vi "task_default.vi"() -> ()   [LabVIEW 2015]
uses:
  Framework/pdbm_test_route/UsrDefine/TaskFeedbackCmd.ctl
  Framework/pdbm_test_route/UsrDefine/TaskReqst.ctl
  Framework/pdbm_tasks/pdbm_tasks.lvlib
  Framework/pdbm_test_route/pdbm_task_route.lvlib
panel:
  in  "error in (no error)":errorcluster
  in  "pdbm_task_data":T1
  # "IMT APPLICATION TASK"
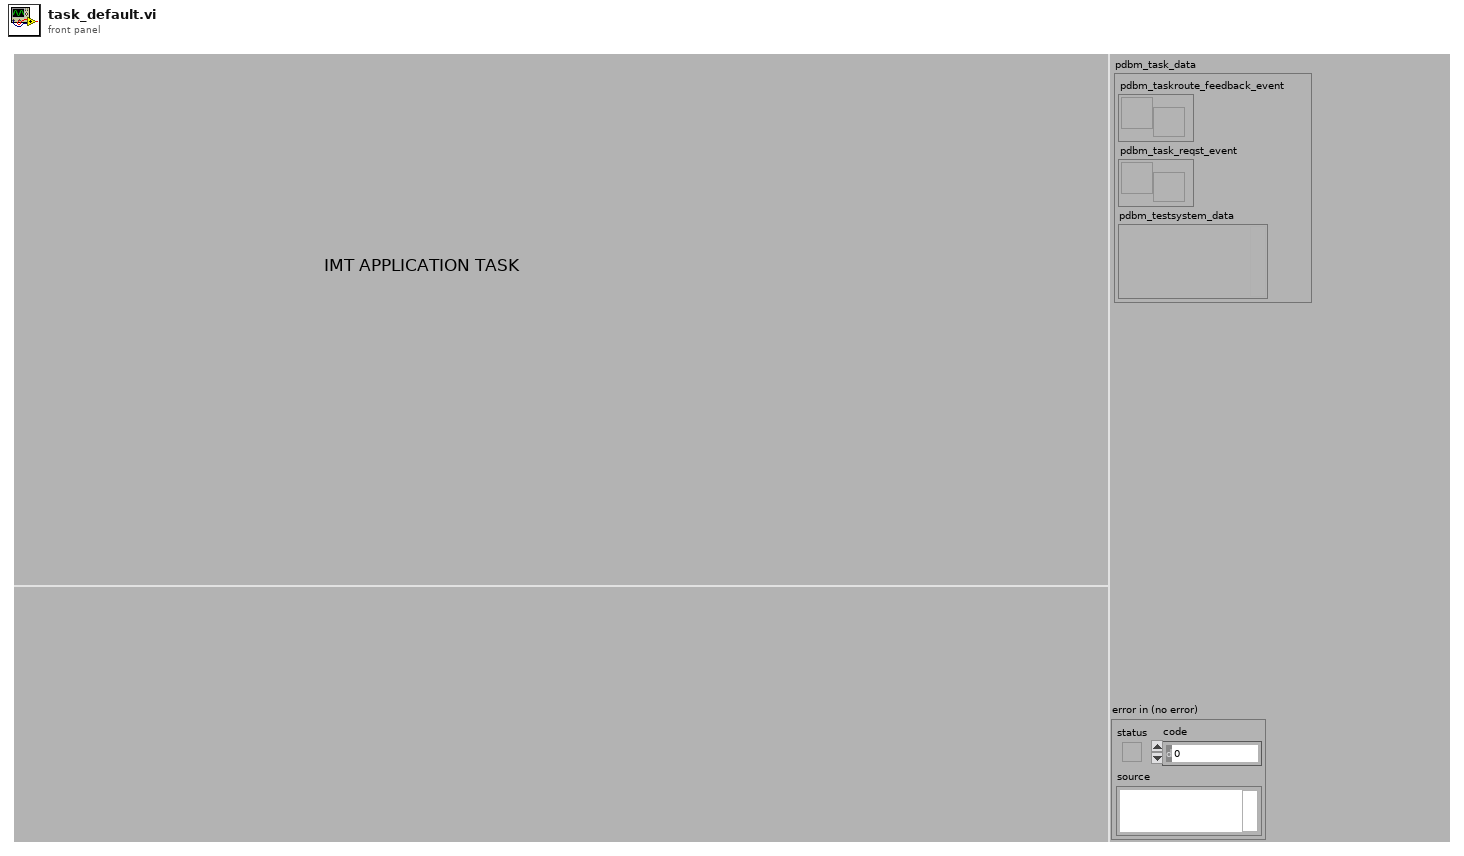
[diagram p1: front panel]
types:
  T1 = cluster{"pdbm_taskroute_feedback_event":refnum<user-event>, "pdbm_task_reqst_event":refnum<user-event>, "pdbm_testsystem_data":variant}
  T2 = typedef "pdbm_tasks.lvlib/PDBM_TestSystem_Data.ctl" = cluster{"pdbm_general_report_info":refnum<vi>, "pdbm_task_progress":refnum<vi>, "pdbm_TestButton":refnum<vi>}
  T3 = cluster{"pdbm_task_reqst_event":refnum<user-event>, "pdbm_taskroute_feedback_event":refnum<user-event>}
  T4 = typedef "pdbm_tasks.lvlib/TaskRequest.ctl" = cluster{"Command":string, "Variant":variant}
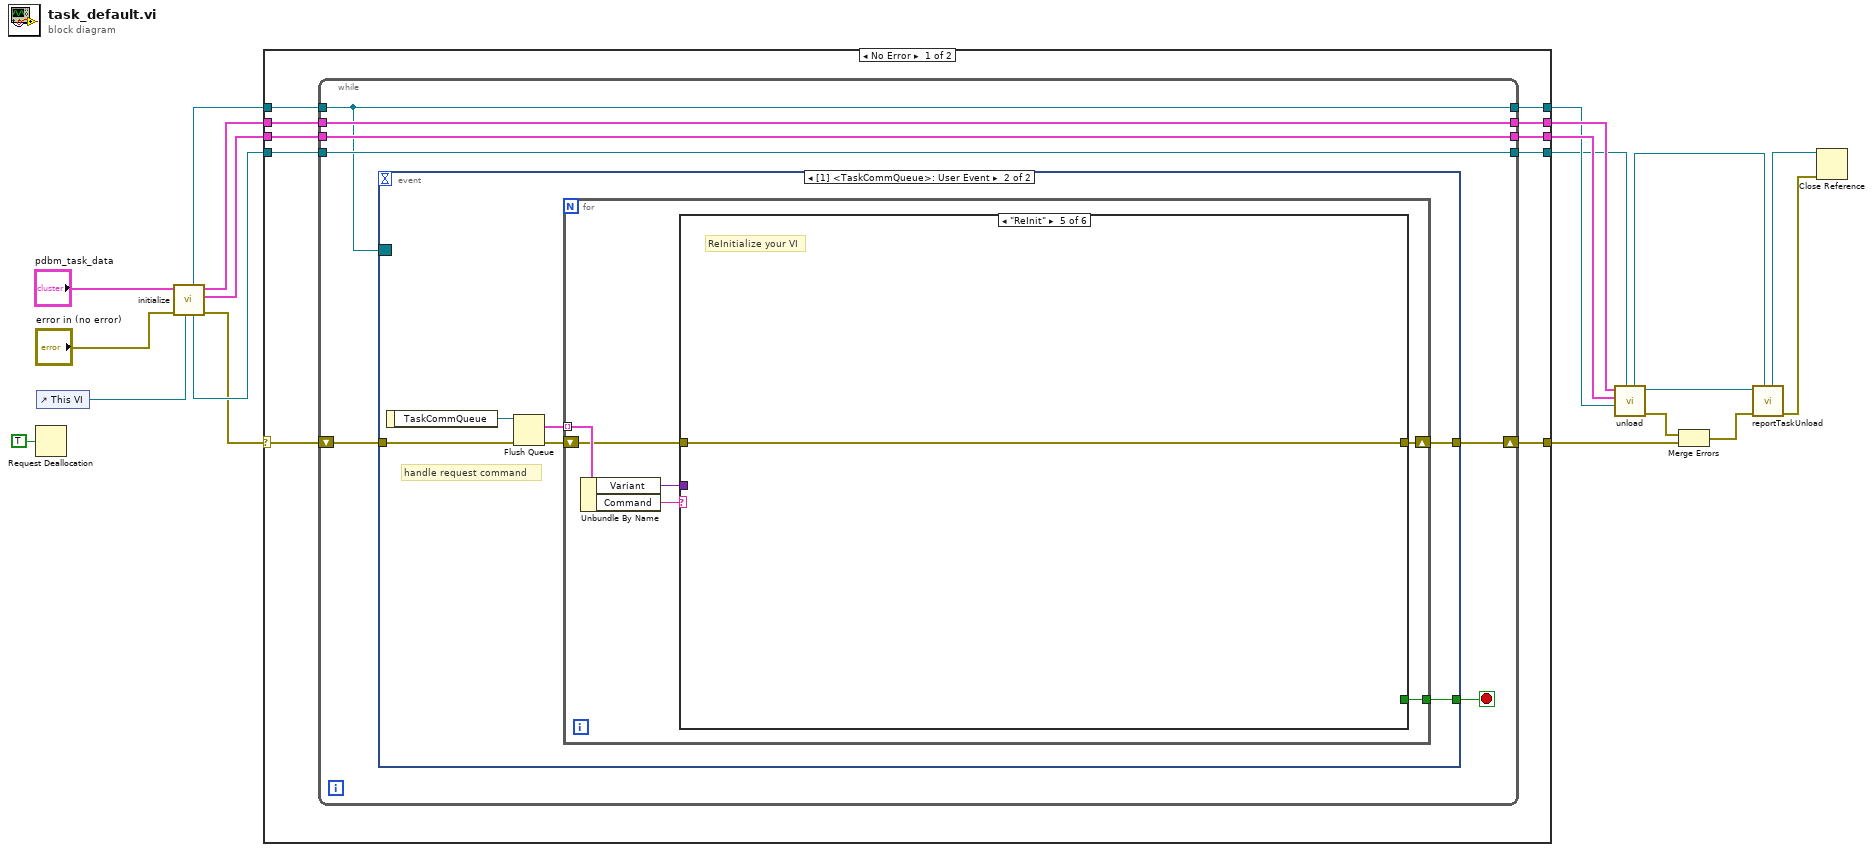
[diagram p0: block diagram]
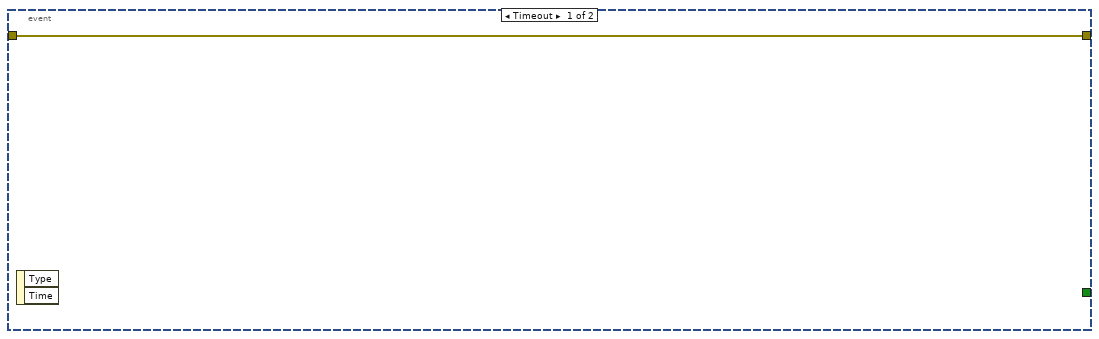
[diagram p2: hidden frame]
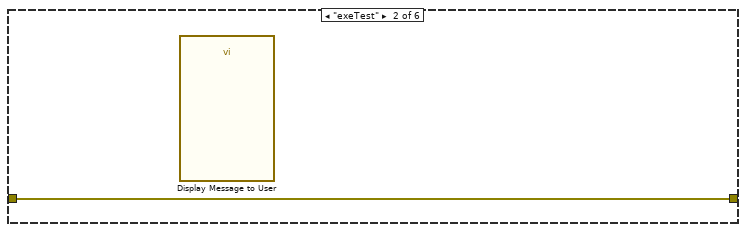
[diagram p4: hidden frame]
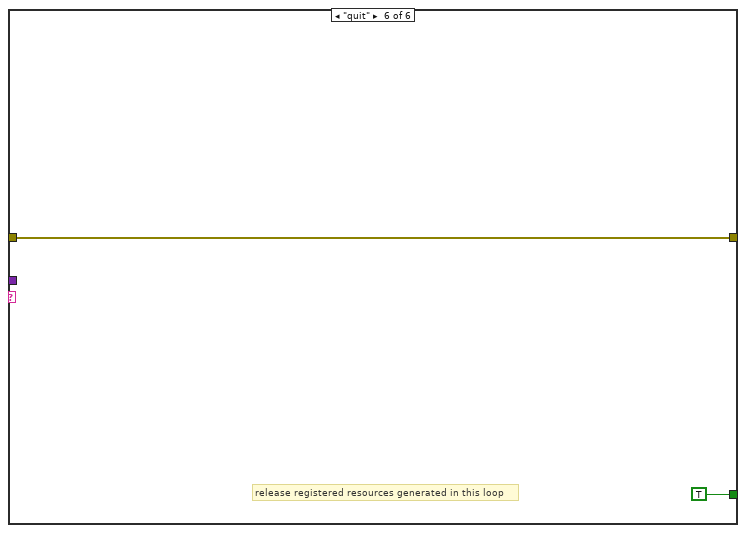
[diagram p7: hidden frame]
diagram:
  n1 = Request Deallocation(TRUE ("flag")) -> ()
  n2 = control-ref of="This VI"() -> (w19:refnum<vi>)
  n3 = call "initialize.vi"("TaskRef in"=w19, "error in"="error in (no error)", "pdbm_task_data"="pdbm_task_data") -> ("error out"=w15:errorcluster, "pdbm_task_data"=w3:T2, "pdbm_task_event"=w16:T3, "TaskRef out"=w17:refnum<vi>, "pdbm_task_reg_reqst_event"=w14:refnum<event-registration>)  [unwired: 4 in]
  n4 = case shown="No Error" w15 {
    selector: w15 -> [w29 w62]
    tunnel: w3 -> [w27 w60]
    tunnel: [w28 w62] -> w10
    tunnel: w17 -> [w22 w59]
    tunnel: w16 -> [w26 w61]
    tunnel: w14 -> [w30 w58]
    tunnel: [w25 w61] -> w13
    tunnel: [w24 w60] -> w12
    tunnel: [w23 w59] -> w2
    tunnel: [w21 w58] -> w11
    frame No Error {
      n5 = while {
        tunnel: w30 -> [w31]
        shift-right: [w36] -> w28
        shift-left: w29 -> [w37]
        tunnel: w22 -> [w32]
        tunnel: w27 -> [w33]
        tunnel: w26 -> [w34]
        tunnel: [w34] -> w25
        tunnel: [w33] -> w24
        tunnel: [w32] -> w23
        tunnel: [w31] -> w21
        stop <- w35 stop-if-true
        n6 = event shown="[1] <TaskCommQueue>: User Event" {
          selector: w31 -> [_ _]
          dyn-events: _ -> [_ _]
          timeout: _ -> [_ _]
          tunnel: w37 -> [w38 w43]
          tunnel: [w38 w40] -> w36
          tunnel: [_ w39] -> w35
          event Timeout {
            n7 = event-data() -> ()  [unwired: 1 in, 2 out]
          }
          event User Event {
            # "handle request command"
            n8 = event-data() -> ("TaskCommQueue"=w44:refnum<queue>)  [unwired: 1 in]
            n9 = Flush Queue(queue=w44, error in (no error)=w43) -> (remaining elements=w41:T4[], error out=w42:errorcluster)  [unwired: 1 out]
            n10 = for {
              tunnel: w41 -> [w50] mode=indexing
              shift-right: [w46] -> w40
              shift-left: w42 -> [w48]
              tunnel: [w45] -> w39
              n11 = Unbundle By Name(w50) -> ("Variant"=w47:variant, "Command"=w49:string)
              n12 = case shown="\"ReInit\"" w49 {
                tunnel: w48 -> [w51 w52 w53 w54 w55 w57]
                tunnel: w47 -> [_ _ _ _ _ _]
                tunnel: [w51 w52 w53 w54 w55 w57] -> w46
                tunnel: [_ _ _ _ _ TRUE] -> w45
                frame "False", Default {
                }
                frame "exeTest" {
                  n13 = call "Display Message to User"() -> ()  [unwired: 10 in, 2 out]
                }
                frame "halt_test" {
                }
                frame "stop_test" {
                }
                frame "ReInit" {
                  # "ReInitialize your VI"
                }
                frame "quit" {
                  # "release registered resources generated in this loop"
                }
              }
            }
          }
        }
      }
    }
    frame Error {
    }
  }
  n14 = call "unload.vi"("TaskRef in"=w2, "pdbm_task_reg_reqst_event"=w11, "pdbm_task_data"=w12, "pdbm_task_event"=w13) -> ("error out"=w9:errorcluster, "pdbm_taskroute_feedback_event"=w8:refnum<user-event>, "TaskRef out"=w1:refnum<vi>)  [unwired: 5 in]
  n15 = Merge Errors(w9, w10) -> (w7:errorcluster)
  n16 = call "reportTaskUnload.vi"("TaskRef"=w1, "error in (no error)"=w7, "pdbm_taskroute_feedback_event"=w8) -> ("error out"=w4:errorcluster, "TaskRef out"=w5:refnum<vi>)  [unwired: 6 in, 1 out]
  n17 = Close Reference(reference=w5, error in (no error)=w4) -> ()  [unwired: 1 out]
